vi "VSG25_Sweep.vi"(3 "Error In":errorcluster, 4 "Sweep Params In":T1={"Start Freq"=0.6, "Stop Freq"=1.0, "Start Hz"=3, "Stop Hz"=3, "Step Freq"=100.0, "Step Hz"=2, "Amplitude"=-10.0, "Dwell Time"=1000.0} {"Start Hz" items=["Hz", "kHz", "MHz", "GHz"]; "Stop Hz" items=["Hz", "kHz", "MHz", "GHz"]; "Step Hz" items=["Hz", "kHz", "MHz", "GHz"]}, 5 "Device Handle In":i32) -> (0 "Error Out":errorcluster, 2 "Device Handle Out":i32)   [LabVIEW 2014]
uses:
  sg_lib/VSG25A.lvlib
  Controls/Frequency Hertz.ctl
  Controls/Sweep Cluster.ctl
panel:
  out "CL Exit":bool
  in  "Run as Subpanel":bool
  out "MSML Exit":bool
  out "Sweep Params Out":T1={"Start Freq"=1.0, "Stop Freq"=2.0, "Start Hz"=3, "Stop Hz"=3, "Step Freq"=100.0, "Step Hz"=2, "Amplitude"=-10.0, "Dwell Time"=100.0} {"Start Hz" items=["Hz", "kHz", "MHz", "GHz"]; "Stop Hz" items=["Hz", "kHz", "MHz", "GHz"]; "Step Hz" items=["Hz", "kHz", "MHz", "GHz"]}
  in  "RF On":bool
  in  "Step Freq Hz":T2 items=["Hz", "kHz", "MHz", "GHz"]
  in  "Stop Freq Hz":T2 items=["Hz", "kHz", "MHz", "GHz"]
  in  "Start Freq Hz":T2 items=["Hz", "kHz", "MHz", "GHz"]
  in  "Amplitude (dBm)":dbl
  out "Sweep Time":dbl
  out "Frequency Span":dbl
  in  "Dwell Time (mS)":dbl
  in  "Step Frequency":dbl
  in  "Stop Frequency":dbl
  in  "Start Frequency":dbl
  # "Step Sweep"
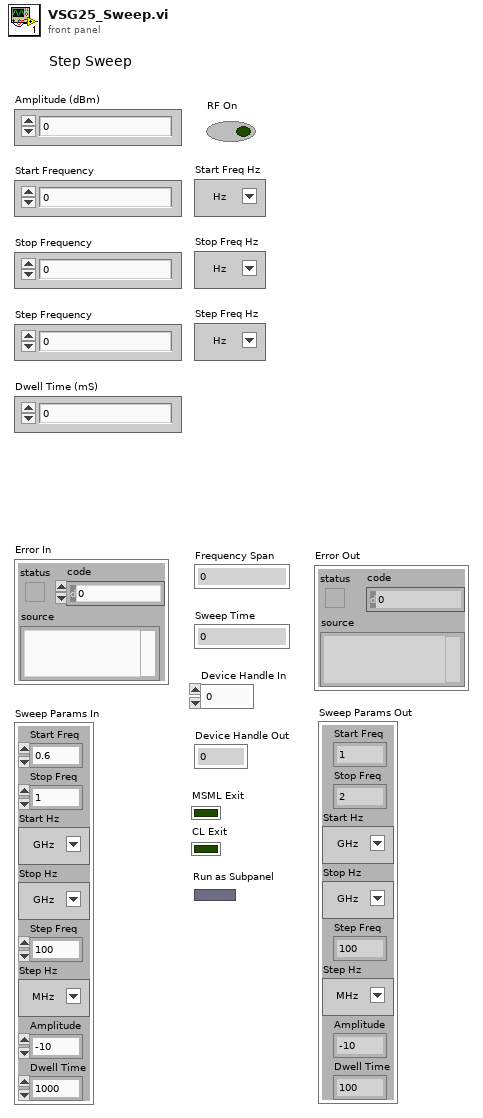
[diagram p1: front panel]
types:
  T1 = typedef "Sweep Cluster.ctl" = cluster{"Start Freq":dbl, "Stop Freq":dbl, "Start Hz":T2, "Stop Hz":T2, "Step Freq":dbl, "Step Hz":T2, "Amplitude":dbl, "Dwell Time":dbl}
  T2 = typedef "Frequency Hertz.ctl" = u16
  T3 = enum32{"Bad", "Idle", "Run top level", "Running"}
  T4 = enum16{"Check Amplitude", "Check Start Freq", "Check Stop Freq", "Check Step Freq", "Check Dwell Time", "Calc Freq Span", "Calc Sweep Time", "Stop RF", "Set Freq And Amp", "Set Sweep", "Finish", ""}
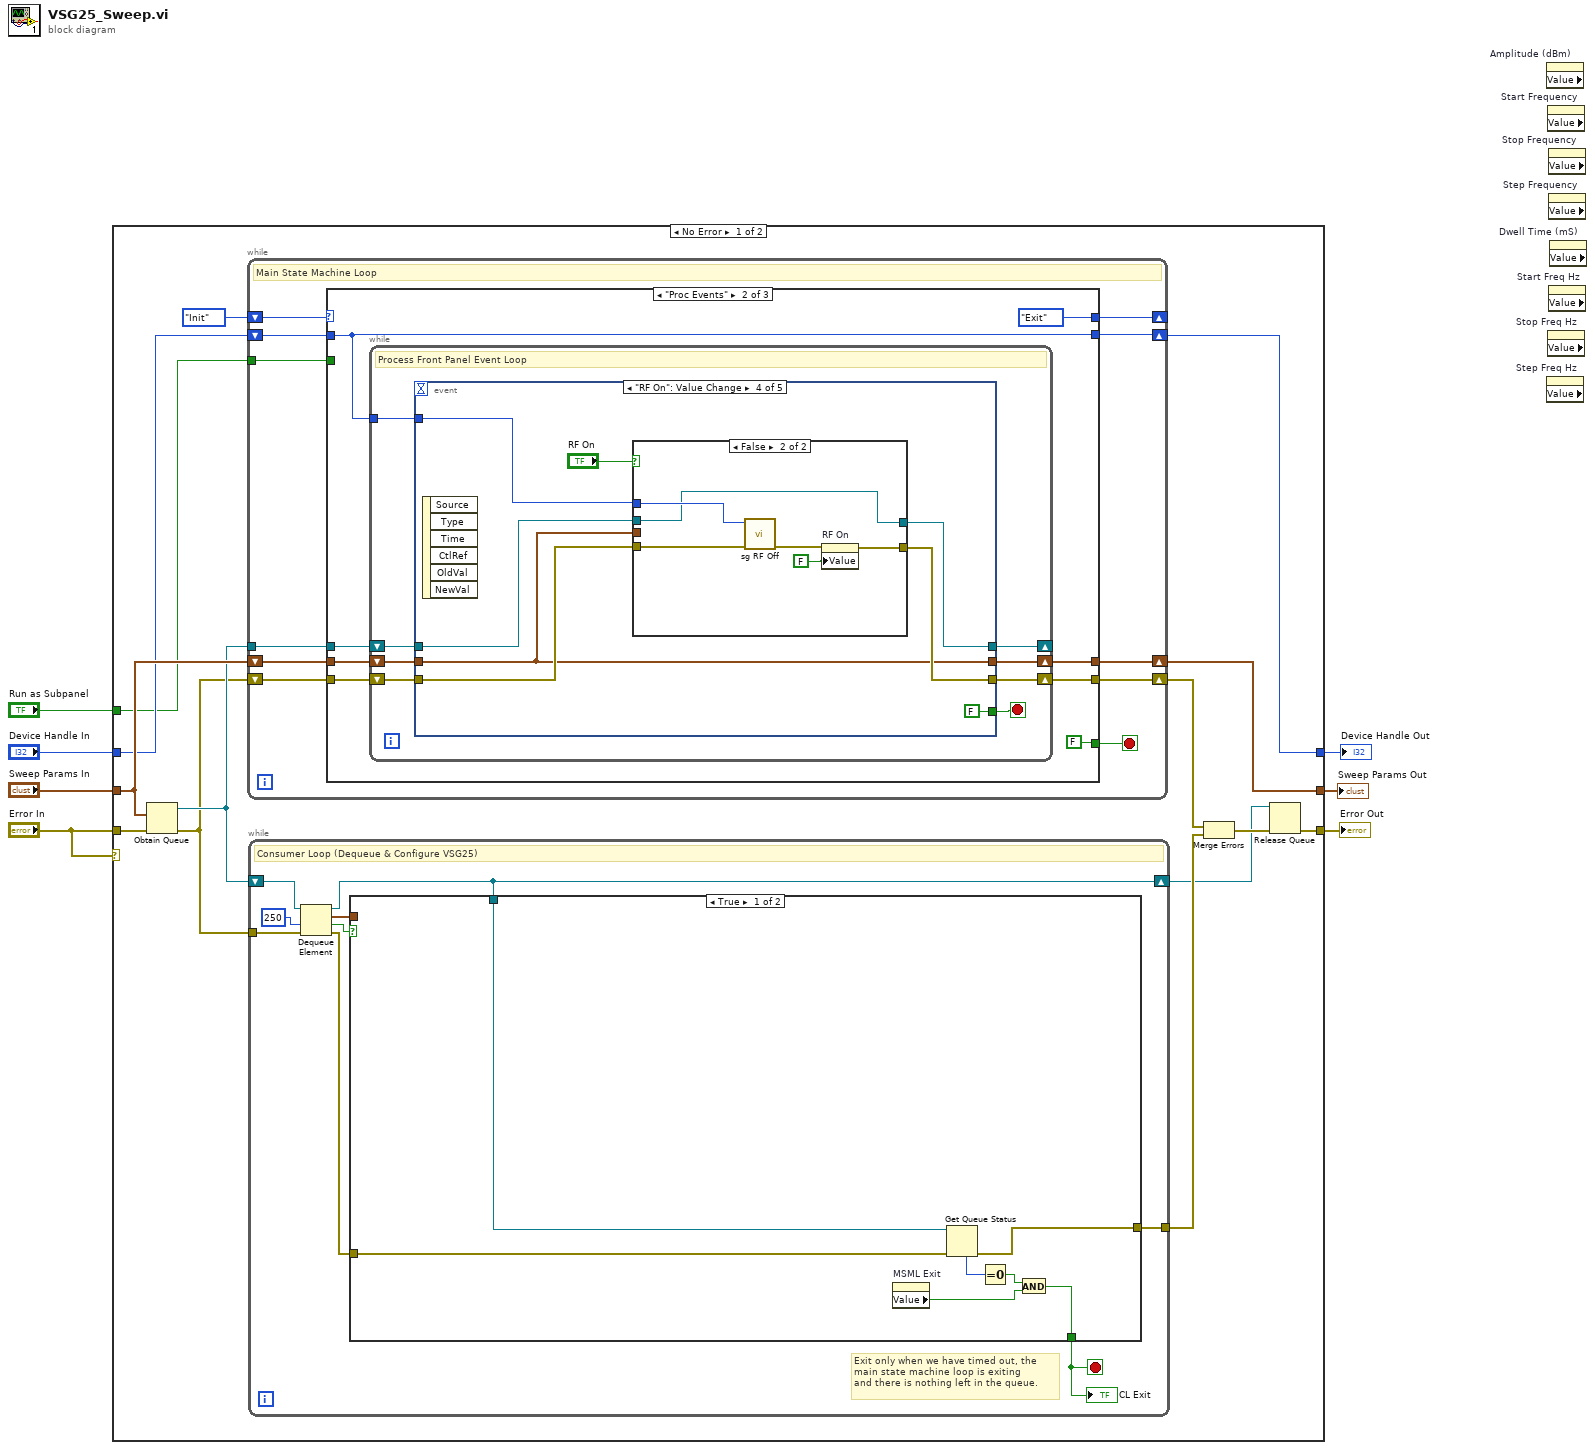
[diagram p0: block diagram]
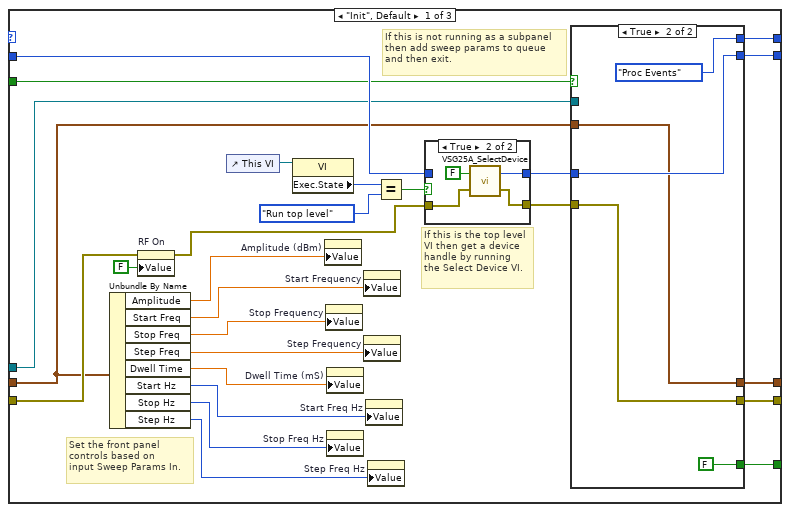
[diagram p2: hidden frame]
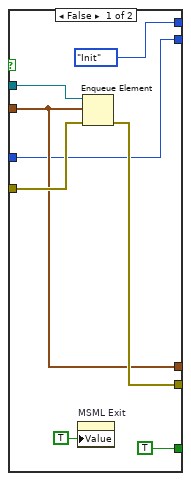
[diagram p3: hidden frame]
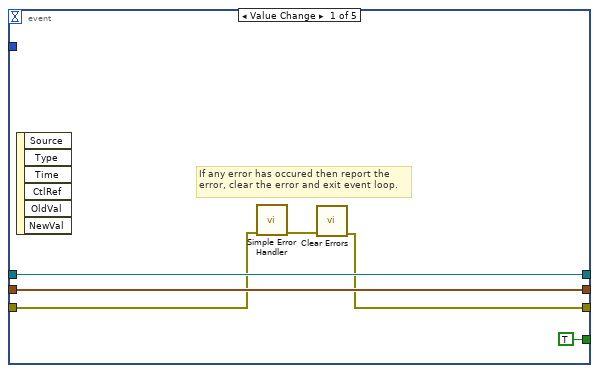
[diagram p5: hidden frame]
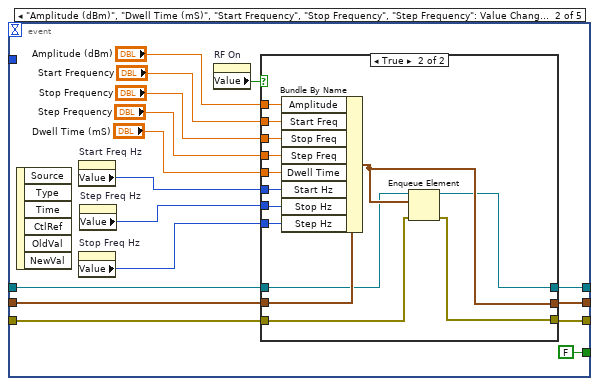
[diagram p6: hidden frame]
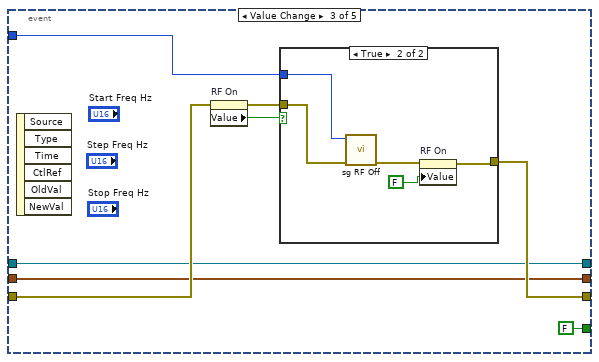
[diagram p8: hidden frame]
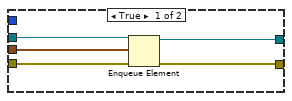
[diagram p10: hidden frame]
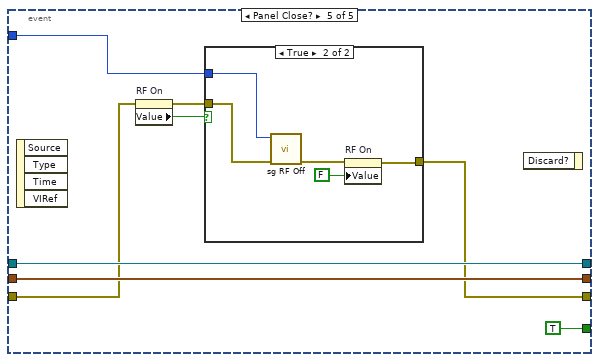
[diagram p11: hidden frame]
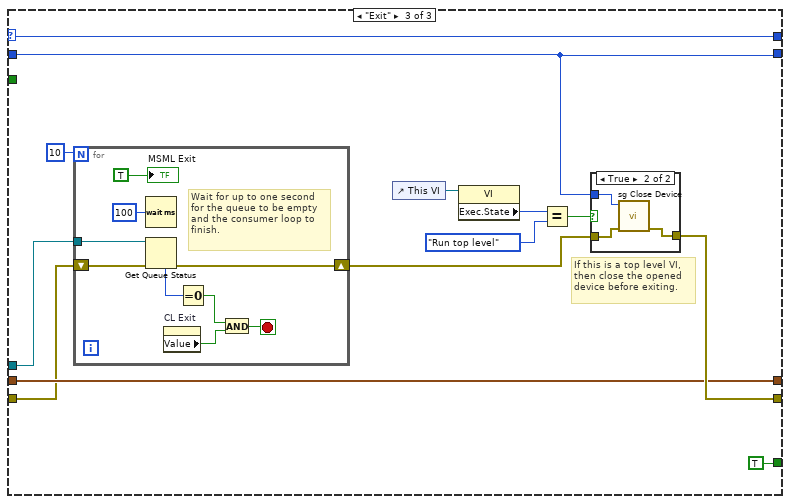
[diagram p13: hidden frame]
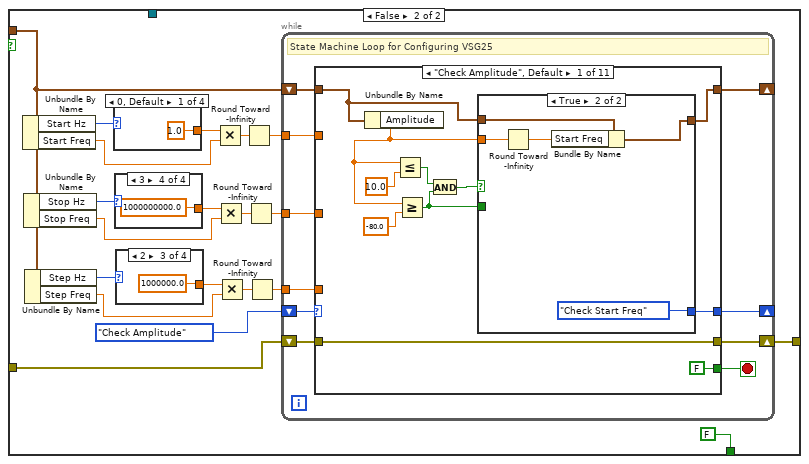
[diagram p15: hidden frame]
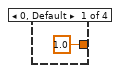
[diagram p16: hidden frame]
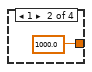
[diagram p17: hidden frame]
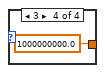
[diagram p18: hidden frame]
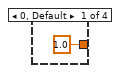
[diagram p19: hidden frame]
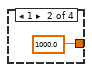
[diagram p20: hidden frame]
diagram:
  n1 = case shown="No Error" "Error In" {
    tunnel: "Error In" -> [w18 w393]
    tunnel: [w19 w393] -> w6
    tunnel: "Sweep Params In" -> [w16 w392]
    tunnel: [w10 w392] -> w4
    tunnel: "Device Handle In" -> [w14 w391]
    tunnel: [w12 w391] -> w2
    tunnel: "Run as Subpanel" -> [w8 _]
    frame No Error {
      n2 = Obtain Queue(element data type=w16, error in (no error)=w18) -> (queue out=w15:refnum<queue>, error out=w11:errorcluster)  [unwired: 3 in, 1 out]
      n3 = while {
        shift-right: [w31] -> _
        shift-left: enum16{"Init", "Proc Events", "Exit"}."Init" -> [w32]
        tunnel: w15 -> [w29]
        shift-right: [w27] -> w12
        shift-left: w14 -> [w28]
        shift-right: [w26] -> w13
        shift-left: w11 -> [w25]
        shift-right: [w24] -> w10
        shift-left: w16 -> [w30]
        tunnel: w8 -> [w22]
        stop <- w23 stop-if-true
        # "Main State Machine Loop"
        n4 = case shown="\"Proc Events\"" w32 {
          selector: w32 -> [_ _ w186]
          tunnel: [w37 enum16{"Init", "Proc Events", "Exit"}."Exit" w186] -> w31
          tunnel: w25 -> [w44 w85 w183]
          tunnel: w30 -> [w40 w84 w185]
          tunnel: w29 -> [w39 w83 w182]
          tunnel: w28 -> [w45 w82 w187]
          tunnel: [w36 w82 w187] -> w27
          tunnel: [w35 w80 w188] -> w26
          tunnel: [w34 w79 w185] -> w24
          tunnel: [w43 FALSE TRUE] -> w23
          tunnel: w22 -> [w41 _ _]
          frame "Init", Default {
            # "If this is not running as a subpanel\nthen add sweep params to queue \nand then exit."
            # "If this is the top level\nVI then get a device\nhandle by running \nthe Select Device VI."
            # "Set the front panel\ncontrols based on \ninput Sweep Params In."
            n5 = Unbundle By Name(w40) -> ("Amplitude"=w57:dbl, "Start Freq"=w56:dbl, "Stop Freq"=w51:dbl, "Step Freq"=w55:dbl, "Dwell Time"=w54:dbl, "Start Hz"=w53:T2, "Stop Hz"=w52:T2, "Step Hz"=w50:T2)
            n6 = property on="RF On" class="Bool (strict)"(error in=w44, "Value"=FALSE ("RF On")) -> (error out=w42:errorcluster)  [unwired: 1 in, 1 out]
            n7 = control-ref of="This VI"() -> (w46:refnum<vi>)
            n8 = property class="VI"(reference=w46) -> ("Exec.State"=w47:T3)  [unwired: 1 in, 2 out]
            n9 = property on="Amplitude (dBm)" class="DigNum (strict)"("Value"=w57) -> ()  [unwired: 2 in, 2 out]
            n10 = property on="Stop Frequency" class="DigNum (strict)"("Value"=w51) -> ()  [unwired: 2 in, 2 out]
            n11 = property on="Dwell Time (mS)" class="DigNum (strict)"("Value"=w54) -> ()  [unwired: 2 in, 2 out]
            n12 = property on="Stop Freq Hz" class="Ring (strict)"("Value"=w52) -> ()  [unwired: 2 in, 2 out]
            n13 = property on="Start Frequency" class="DigNum (strict)"("Value"=w56) -> ()  [unwired: 2 in, 2 out]
            n14 = property on="Step Frequency" class="DigNum (strict)"("Value"=w55) -> ()  [unwired: 2 in, 2 out]
            n15 = property on="Start Freq Hz" class="Ring (strict)"("Value"=w53) -> ()  [unwired: 2 in, 2 out]
            n16 = property on="Step Freq Hz" class="Ring (strict)"("Value"=w50) -> ()  [unwired: 2 in, 2 out]
            n17 = Equal?(x=w47, y=T3."Run top level" ("Execution:State 2")) -> (x = y?=w49:bool)
            n18 = case shown="True" w49 {
              tunnel: [w73 w77] -> w33
              tunnel: w45 -> [w73 _]
              tunnel: w42 -> [w72 w75]
              tunnel: [w72 w74] -> w38
              frame False {
              }
              frame True {
                n19 = call "VSG25A_SelectDevice.vi"("ErrorIn"=w75, "AutoSel"=FALSE) -> ("ErrorOut"=w74:errorcluster, "deviceHandle"=w77:i32)
              }
            }
            n20 = case shown="True" w41 {
              tunnel: [TRUE FALSE] -> w43
              tunnel: w40 -> [w61 w68]
              tunnel: w39 -> [w65 _]
              tunnel: w38 -> [w64 w67]
              tunnel: [enum16{"Init", "Proc Events", "Exit"}."Init" enum16{"Init", "Proc Events", "Exit"}."Proc Events"] -> w37
              tunnel: [w60 w69] -> w36
              tunnel: [w62 w67] -> w35
              tunnel: [w61 w68] -> w34
              tunnel: w33 -> [w60 w69]
              frame False {
                n21 = property on="MSML Exit" class="Bool (strict)"("Value"=TRUE ("MSML Exit")) -> ()  [unwired: 2 in, 2 out]
                n22 = Enqueue Element(queue=w65, element=w61, error in (no error)=w64) -> (error out=w62:errorcluster)  [unwired: 1 in, 2 out]
              }
              frame True {
              }
            }
          }
          frame "Proc Events" {
            n23 = while {
              shift-right: [w91] -> w79
              shift-left: w84 -> [w92]
              shift-right: [w90] -> w80
              shift-left: w85 -> [w93]
              shift-right: [w88] -> _
              shift-left: w83 -> [w89]
              tunnel: w82 -> [w87]
              stop <- w86 stop-if-true
              # "Process Front Panel Event Loop"
              n24 = event shown="[3] \"RF On\": Value Change" {
                selector: _ -> [_ _ _ _ _]
                dyn-events: _ -> [_ _ _ _ _]
                timeout: _ -> [_ _ _ _ _]
                tunnel: w93 -> [w96 w104 w137 w151 w167]
                tunnel: w92 -> [w98 w113 w135 w150 w172]
                tunnel: [w98 w114 w135 w150 w172] -> w91
                tunnel: [w94 w103 w140 w154 w166] -> w90
                tunnel: w89 -> [w99 w102 w134 w152 w171]
                tunnel: [w99 w101 w134 w149 w171] -> w88
                tunnel: w87 -> [_ _ w136 w148 w168]
                tunnel: [TRUE FALSE FALSE FALSE TRUE] -> w86
                event "Error In.status": Value Change {
                  # "If any error has occured then report the \nerror, clear the error and exit event loop."
                  n25 = event-data() -> ()  [unwired: 1 in, 6 out]
                  n26 = call <vilib>:"Simple Error Handler.vi"("error in (no error)"=w96) -> ("error out"=w95:errorcluster)  [unwired: 4 in, 4 out]
                  n27 = call <vilib>:"Clear Errors.vi"("error in (no error)"=w95) -> ("error out"=w94:errorcluster)  [unwired: 5 in, 1 out]
                }
                event "Amplitude (dBm)", "Dwell Time (mS)", "Start Frequency", "Stop Frequency", "Step Frequency": Value Change {
                  n28 = event-data() -> ()  [unwired: 1 in, 6 out]
                  n29 = property on="Start Freq Hz" class="Ring (strict)"() -> ("Value"=w107:T2)  [unwired: 2 in, 2 out]
                  n30 = property on="Stop Freq Hz" class="Ring (strict)"() -> ("Value"=w105:T2)  [unwired: 2 in, 2 out]
                  n31 = property on="Step Freq Hz" class="Ring (strict)"() -> ("Value"=w106:T2)  [unwired: 2 in, 2 out]
                  n32 = property on="RF On" class="Bool (strict)"() -> ("Value"=w115:bool)  [unwired: 2 in, 2 out]
                  n33 = case shown="True" w115 {
                    tunnel: [w117 w123] -> w114
                    tunnel: w113 -> [w117 w132]
                    tunnel: "Amplitude (dBm)" -> [_ w131]
                    tunnel: "Start Frequency" -> [_ w130]
                    tunnel: "Stop Frequency" -> [_ w129]
                    tunnel: "Step Frequency" -> [_ w128]
                    tunnel: "Dwell Time (mS)" -> [_ w127]
                    tunnel: w107 -> [_ w126]
                    tunnel: w106 -> [_ w125]
                    tunnel: w105 -> [_ w124]
                    tunnel: w104 -> [w116 w122]
                    tunnel: [w116 w121] -> w103
                    tunnel: w102 -> [w118 w120]
                    tunnel: [w118 w119] -> w101
                    frame False {
                    }
                    frame True {
                      n34 = Bundle By Name(cluster=w132, "Amplitude"=w131, "Start Freq"=w130, "Stop Freq"=w129, "Step Freq"=w128, "Dwell Time"=w127, "Start Hz"=w126, "Stop Hz"=w125, "Step Hz"=w124) -> (w123:T1)
                      n35 = Enqueue Element(queue=w120, element=w123, error in (no error)=w122) -> (queue out=w119:refnum<queue>, error out=w121:errorcluster)  [unwired: 1 in, 1 out]
                    }
                  }
                }
                event Value Change {
                  n36 = event-data() -> ()  [unwired: 1 in, 6 out]
                  n37 = property on="RF On" class="Bool (strict)"(error in=w137) -> (error out=w138:errorcluster, "Value"=w139:bool)  [unwired: 1 in, 1 out]
                  n38 = case shown="True" w139 {
                    tunnel: [w141 w144] -> w140
                    tunnel: w138 -> [w141 w143]
                    tunnel: w136 -> [_ w142]
                    frame False {
                    }
                    frame True {
                      n39 = call "sg RF Off.vi"("error in (no error)"=w143, "device"=w142) -> ("error out"=w145:errorcluster)  [unwired: 8 in, 1 out]
                      n40 = property on="RF On" class="Bool (strict)"(error in=w145, "Value"=FALSE ("RF On")) -> (error out=w144:errorcluster)  [unwired: 1 in, 1 out]
                    }
                  }
                }
                event "RF On": Value Change {
                  n41 = event-data() -> ()  [unwired: 1 in, 6 out]
                  n42 = case shown="False" "RF On" {
                    tunnel: [w155 w163] -> w154
                    tunnel: w152 -> [w159 w160]
                    tunnel: w150 -> [w158 _]
                    tunnel: w151 -> [w157 w162]
                    tunnel: [w156 w160] -> w149
                    tunnel: w148 -> [_ w161]
                    frame True {
                      n43 = Enqueue Element(queue=w159, element=w158, error in (no error)=w157) -> (queue out=w156:refnum<queue>, error out=w155:errorcluster)  [unwired: 1 in, 1 out]
                    }
                    frame False {
                      n44 = call "sg RF Off.vi"("error in (no error)"=w162, "device"=w161) -> ("error out"=w164:errorcluster)  [unwired: 8 in, 1 out]
                      n45 = property on="RF On" class="Bool (strict)"(error in=w164, "Value"=FALSE ("RF On")) -> (error out=w163:errorcluster)  [unwired: 1 in, 1 out]
                    }
                  }
                }
                event Panel Close? {
                  n46 = event-data() -> ()  [unwired: 1 in, 4 out]
                  n47 = property on="RF On" class="Bool (strict)"(error in=w167) -> (error out=w169:errorcluster, "Value"=w170:bool)  [unwired: 1 in, 1 out]
                  n48 = case shown="True" w170 {
                    tunnel: [w174 w177] -> w166
                    tunnel: w169 -> [w174 w176]
                    tunnel: w168 -> [_ w175]
                    frame False {
                    }
                    frame True {
                      n49 = call "sg RF Off.vi"("error in (no error)"=w176, "device"=w175) -> ("error out"=w178:errorcluster)  [unwired: 8 in, 1 out]
                      n50 = property on="RF On" class="Bool (strict)"(error in=w178, "Value"=FALSE ("RF On")) -> (error out=w177:errorcluster)  [unwired: 1 in, 1 out]
                    }
                  }
                  n51 = event-data() -> ()  [unwired: 2 in, 1 out]
                }
              }
            }
          }
          frame "Exit" {
            # "If this is a top level VI, \nthen close the opened \ndevice before exiting."
            n52 = for {
              N: 10 -> [_]
              tunnel: w182 -> [w199]
              shift-right: [w198] -> w181
              shift-left: w183 -> [w200]
              stop <- w195 stop-if-true
              # "Wait for up to one second\nfor the queue to be empty\nand the consumer loop to\nfinish."
              n53 = Wait (ms)(milliseconds to wait=u32 100) -> ()  [unwired: 1 out]
              n54 = Get Queue Status(queue=w199, error in (no error)=w200) -> (error out=w198:errorcluster, # elements in queue=w197:i32)  [unwired: 1 in, 6 out]
              n55 = property on="CL Exit" class="Bool (strict)"() -> ("Value"=w194:bool)  [unwired: 2 in, 2 out]
              n56 = Equal To 0?(x=w197) -> (x = 0?=w193:bool)
              n57 = And(x=w193, y=w194) -> (x .and. y?=w195:bool)
              "MSML Exit" <- TRUE
            }
            n58 = control-ref of="This VI"() -> (w192:refnum<vi>)
            n59 = property class="VI"(reference=w192) -> ("Exec.State"=w191:T3)  [unwired: 1 in, 2 out]
            n60 = Equal?(x=w191, y=T3."Run top level" ("Execution:State 2")) -> (x = y?=w189:bool)
            n61 = case shown="True" w189 {
              tunnel: w187 -> [_ w205]
              tunnel: w181 -> [w202 w204]
              tunnel: [w202 w203] -> w188
              frame False {
              }
              frame True {
                n62 = call "sg Close Device.vi"("error in (no error)"=w204, "device"=w205) -> ("error out"=w203:errorcluster)  [unwired: 8 in, 1 out]
              }
            }
          }
        }
      }
      n63 = while {
        tunnel: w11 -> [w214]
        shift-right: [w206] -> w9
        shift-left: w15 -> [w213]
        tunnel: [w211] -> w21
        stop <- w207 stop-if-true
        # "Exit only when we have timed out, the \nmain state machine loop is exiting \nand there is nothing left in the queue."
        # "Consumer Loop (Dequeue & Configure VSG25)"
        n64 = Dequeue Element(queue=w213, timeout in ms (-1)=250, error in (no error)=w214) -> (queue out=w206:refnum<queue>, element=w212:T1, timed out?=w209:bool, error out=w208:errorcluster)
        n65 = case shown="True" w209 {
          tunnel: w212 -> [_ w225]
          tunnel: [w217 w224] -> w211
          tunnel: w208 -> [w221 w223]
          tunnel: [w216 FALSE] -> w207
          tunnel: w206 -> [w215 _]
          frame True {
            n66 = property on="MSML Exit" class="Bool (strict)"() -> ("Value"=w218:bool)  [unwired: 2 in, 2 out]
            n67 = Get Queue Status(queue=w215, error in (no error)=w221) -> (error out=w217:errorcluster, # elements in queue=w220:i32)  [unwired: 1 in, 6 out]
            n68 = Equal To 0?(x=w220) -> (x = 0?=w219:bool)
            n69 = And(x=w219, y=w218) -> (x .and. y?=w216:bool)
          }
          frame False {
            n70 = Unbundle By Name(w225) -> ("Start Hz"=w238:T2, "Start Freq"=w239:dbl)
            n71 = Unbundle By Name(w225) -> ("Stop Hz"=w237:T2, "Stop Freq"=w236:dbl)
            n72 = Unbundle By Name(w225) -> ("Step Hz"=w229:T2, "Step Freq"=w230:dbl)
            n73 = case shown="0, Default" w238 {
              tunnel: [1.0 ("y") 1000.0 ("y") 1000000.0 ("y") 1000000000.0 ("y")] -> w240
              frame 0, Default {
              }
              frame 1 {
              }
              frame 2 {
              }
              frame 3 {
              }
            }
            n74 = case shown="3" w237 {
              tunnel: [1.0 ("y") 1000.0 ("y") 1000000.0 ("y") 1000000000.0 ("y")] -> w235
              frame 0, Default {
              }
              frame 1 {
              }
              frame 2 {
              }
              frame 3 {
              }
            }
            n75 = case shown="2" w229 {
              tunnel: [1.0 ("y") 1000.0 ("y") 1000000.0 ("y") 1000000000.0 ("y")] -> w231
              frame 0, Default {
              }
              frame 1 {
              }
              frame 2 {
              }
              frame 3 {
              }
            }
            n76 = Multiply(x=w240, y=w239) -> (x*y=w234:dbl)
            n77 = Multiply(x=w235, y=w236) -> (x*y=w233:dbl)
            n78 = Multiply(x=w231, y=w230) -> (x*y=w232:dbl)
            n79 = Round Toward -Infinity(1:w234) -> (0:w228:dbl)
            n80 = Round Toward -Infinity(1:w233) -> (0:w227:dbl)
            n81 = Round Toward -Infinity(1:w232) -> (0:w226:dbl)
            n82 = while {
              shift-right: [w261] -> _
              shift-left: w225 -> [w262]
              shift-right: [w260] -> _
              shift-left: T4."Check Amplitude" -> [w263]
              tunnel: w228 -> [w259]
              tunnel: w227 -> [w258]
              tunnel: w226 -> [w257]
              shift-right: [w255] -> w224
              shift-left: w223 -> [w256]
              stop <- w254 stop-if-true
              # "State Machine Loop for Configuring VSG25"
              n83 = case shown="\"Check Amplitude\", Default" w263 {
                selector: w263 -> [_ _ _ _ _ _ _ _ _ _ w384]
                tunnel: w262 -> [w268 w289 w307 w320 w333 w343 w353 w358 w365 w373 w379]
                tunnel: [w267 w289 w307 w320 w333 w343 w353 w358 w365 w373 w379] -> w261
                tunnel: [w266 w297 w308 w321 w334 T4."Calc Sweep Time" T4."Stop RF" T4."Set Freq And Amp" T4."Set Sweep" T4."Finish" w384] -> w260
                tunnel: w259 -> [_ w295 _ _ _ w346 _ _ _ _ _]
                tunnel: w258 -> [_ w300 w312 _ _ w347 _ _ _ _ _]
                tunnel: w257 -> [_ w299 _ w322 _ _ _ _ _ _ _]
                tunnel: w256 -> [w265 w290 w306 w319 w332 w342 w352 w360 w369 w377 w383]
                tunnel: [w265 w290 w306 w319 w332 w342 w352 w359 w368 w376 w381] -> w255
                tunnel: [FALSE FALSE FALSE FALSE FALSE FALSE FALSE FALSE FALSE FALSE TRUE] -> w254
                frame "Check Amplitude", Default {
                  n84 = Unbundle By Name(w268) -> ("Amplitude"=w269:dbl)
                  n85 = Less Or Equal?(x=w269, y=10.0) -> (x <= y?=w273:bool)
                  n86 = Greater Or Equal?(x=w269, y=-80.0) -> (x >= y?=w270:bool)
                  n87 = And(x=w273, y=w270) -> (x .and. y?=w274:bool)
                  n88 = case shown="True" w274 {
                    tunnel: w270 -> [w282 _]
                    tunnel: w269 -> [_ w286]
                    tunnel: w268 -> [w279 w285]
                    tunnel: [w278 w284] -> w267
                    tunnel: [T4."Finish" T4."Check Start Freq"] -> w266
                    frame False {
                      n89 = Select(t=10.0, s=w282, f=-80.0) -> (s? t:f=w277:dbl)
                      n90 = Bundle By Name(cluster=w279, "Start Freq"=w277) -> (w278:T1)
                      n91 = property on="Amplitude (dBm)" class="DigNum (strict)"("Value"=w277) -> ()  [unwired: 2 in, 2 out]
                      n92 = One Button Dialog(message="Invalid Amplitude.\nValue must be between\n-80 dBm and 10 dBm.") -> ()  [unwired: 1 in, 1 out]
                    }
                    frame True {
                      n93 = Round Toward -Infinity(1:w286) -> (0:w287:dbl)
                      n94 = Bundle By Name(cluster=w285, "Start Freq"=w287) -> (w284:T1)
                    }
                  }
                }
                frame "Check Start Freq" {
                  n95 = Subtract(x=w300, y=w299) -> (x-y=w298:dbl)
                  n96 = Greater Or Equal?(x=w295, y=80000000.0) -> (x >= y?=w293:bool)
                  n97 = Less Or Equal?(x=w295, y=w298) -> (x <= y?=w292:bool)
                  n98 = Less Or Equal?(x=w295, y=2500000000.0) -> (x <= y?=w291:bool)
                  n99 = Compound Arithmetic op=AND(w293, w292, w291) -> (w294:bool)
                  n100 = case shown="True" w294 {
                    tunnel: [T4."Finish" T4."Check Stop Freq"] -> w297
                    frame False {
                      n101 = One Button Dialog(message="Start frequency must \nbe greater than 80 MHz,\nless than 2.5 GHz and \nless than stop frequency \nby one step.") -> ()  [unwired: 1 in, 1 out]
                    }
                    frame True {
                    }
                  }
                }
                frame "Check Stop Freq" {
                  n102 = Greater Or Equal?(x=w312, y=80000000.0) -> (x >= y?=w311:bool)
                  n103 = Less Or Equal?(x=w312, y=2500000000.0) -> (x <= y?=w310:bool)
                  n104 = Compound Arithmetic op=AND(w311, w310) -> (w309:bool)
                  n105 = case shown="True" w309 {
                    tunnel: [T4."Finish" T4."Check Step Freq"] -> w308
                    frame False {
                      n106 = One Button Dialog(message="Stop frequency must \nbe greater than 80 MHz,\nand less than 2.5 GHz.") -> ()  [unwired: 1 in, 1 out]
                    }
                    frame True {
                    }
                  }
                }
                frame "Check Step Freq" {
                  n107 = Greater Or Equal?(x=w322, y=80000000.0) -> (x >= y?=w325:bool)
                  n108 = Less Or Equal?(x=w322, y=2500000000.0) -> (x <= y?=w324:bool)
                  n109 = Compound Arithmetic op=AND(w325, w324) -> (w323:bool)
                  n110 = case shown="True" w323 {
                    tunnel: [T4."Finish" T4."Check Dwell Time"] -> w321
                    frame False {
                      n111 = One Button Dialog(message="Step frequency must \nbe greater than 80 MHz,\nand less than 2.5 GHz.") -> ()  [unwired: 1 in, 1 out]
                    }
                    frame True {
                    }
                  }
                }
                frame "Check Dwell Time" {
                  n112 = Unbundle By Name(w333) -> ("Dwell Time"=w337:dbl)
                  n113 = Greater Or Equal?(x=w337, y=1.0) -> (x >= y?=w335:bool)
                  n114 = case shown="True" w335 {
                    tunnel: [T4."Finish" T4."Calc Freq Span"] -> w334
                    frame False {
                      n115 = One Button Dialog(message="Dwell time must be greater \nthan 1 milliSecond.") -> ()  [unwired: 1 in, 1 out]
                    }
                    frame True {
                    }
                  }
                }
                frame "Calc Freq Span" {
                  n116 = Subtract(x=w347, y=w346) -> (x-y=→"Frequency Span":dbl)
                }
                frame "Calc Sweep Time" {
                  n117 = Unbundle By Name(w353) -> ("Dwell Time"=w351:dbl)
                  n118 = Divide(x=w351, y=1000.0) -> (x/y=w349:dbl)
                  n119 = Round Toward -Infinity(1:w349) -> (0:→"Sweep Time":dbl)
                }
                frame "Stop RF" {
                  n120 = property on="Device Handle In" class="DigNum (strict)"() -> ("Value"=w357:i32)  [unwired: 2 in, 2 out]
                  n121 = call "sg RF Off.vi"("error in (no error)"=w360, "device"=w357) -> ("error out"=w359:errorcluster)  [unwired: 8 in, 1 out]
                }
                frame "Set Freq And Amp" {
                  n122 = Unbundle By Name(w365) -> ("Amplitude"=w367:dbl)
                  n123 = property on="Device Handle In" class="DigNum (strict)"() -> ("Value"=w363:i32)  [unwired: 2 in, 2 out]
                  n124 = call "sg Set Frequency Amplitude.vi"("error in (no error)"=w369, "amplitude"=w367, "frequency"=800000000.0, "device"=w363) -> ("error out"=w368:errorcluster)  [unwired: 6 in, 1 out]
                }
                frame "Set Sweep" {
                  n125 = property on="Sweep Time" class="DigNum (strict)" props=["Value"]() -> ()  [unwired: 2 in, 3 out]
                  n126 = property on="Frequency Span" class="DigNum (strict)"() -> ("Value"=w375:dbl)  [unwired: 2 in, 2 out]
                  n127 = property on="Device Handle In" class="DigNum (strict)"() -> ("Value"=w371:i32)  [unwired: 2 in, 2 out]
                  n128 = call "sg Set Sweep.vi"("error in (no error)"=w377, "span"=5.0, "time"=w375, "device"=w371) -> ("error out"=w376:errorcluster)  [unwired: 6 in, 1 out]
                }
                frame "Finish" {
                  n129 = case shown="No Error" w383 {
                    selector: w383 -> [w386 w387]
                    tunnel: [w386 w389] -> w382
                    tunnel: [TRUE FALSE] -> w380
                    frame No Error {
                    }
                    frame Error {
                      n130 = call <vilib>:"Simple Error Handler.vi"("error in (no error)"=w387) -> ("error out"=w388:errorcluster)  [unwired: 4 in, 4 out]
                      n131 = call <vilib>:"Clear Errors.vi"("error in (no error)"=w388) -> ("error out"=w389:errorcluster)  [unwired: 5 in, 1 out]
                    }
                  }
                  n132 = property on="RF On" class="Bool (strict)"(error in=w382, "Value"=w380) -> (error out=w381:errorcluster)  [unwired: 1 in, 1 out]
                }
              }
            }
          }
        }
        "CL Exit" <- w207
      }
      n133 = Merge Errors(w13, w21) -> (w20:errorcluster)
      n134 = Release Queue(queue=w9, error in (no error)=w20) -> (error out=w19:errorcluster)  [unwired: 1 in, 2 out]
    }
    frame Error {
    }
  }
  "Error Out" <- w6
  "Device Handle Out" <- w2
  "Sweep Params Out" <- w4
  n135 = property on="Amplitude (dBm)" class="DigNum (strict)" props=["Value"]() -> ()  [unwired: 2 in, 3 out]
  n136 = property on="Step Freq Hz" class="Ring (strict)" props=["Value"]() -> ()  [unwired: 2 in, 3 out]
  n137 = property on="Start Frequency" class="DigNum (strict)" props=["Value"]() -> ()  [unwired: 2 in, 3 out]
  n138 = property on="Stop Freq Hz" class="Ring (strict)" props=["Value"]() -> ()  [unwired: 2 in, 3 out]
  n139 = property on="Stop Frequency" class="DigNum (strict)" props=["Value"]() -> ()  [unwired: 2 in, 3 out]
  n140 = property on="Step Frequency" class="DigNum (strict)" props=["Value"]() -> ()  [unwired: 2 in, 3 out]
  n141 = property on="Start Freq Hz" class="Ring (strict)" props=["Value"]() -> ()  [unwired: 2 in, 3 out]
  n142 = property on="Dwell Time (mS)" class="DigNum (strict)" props=["Value"]() -> ()  [unwired: 2 in, 3 out]
